vi "PDash Duplicate Module.vi"(8 "error in":errorcluster, 10 "Current Selection":T1, 11 "Project":refnum<class "Project.lvclass">) -> (0 "error out":errorcluster)   [LabVIEW 2020, in "Panther Dashboard.lvlib"]
doc: "Panther Dashboard DQMH UI Template"
uses:
  Panther Dashboard.lvlib
  Class/Project/Project.lvclass
  Class/Library/Library.lvclass
  C:/GitClones/PantherLAB/PantherDashboard/src/LabVIEW/Panther Dashboard/Class/LabVIEWItem/LabVIEWItem.lvclass
  Class/VI/VI.lvclass
  Class/Library/Library.lvclass/Library.ctl
  Class/LabVIEWItem/LabVIEWItem.lvclass/LabVIEWItem.ctl
  Class/Project/Project.lvclass/Project.ctl
  <vilib>/Delacor/Delacor QMH/Libraries/_Scripting Support/Module Type--enum.ctl
  <vilib>/Delacor/Delacor QMH/Libraries/_Scripting Support/dqmh_lib_DQMH Scripting Support.lvlib
  <vilib>/Delacor/Delacor QMH/Libraries/_Scripting Support/Module Info--cluster.ctl
  Controls/Cancel.ctl
  Controls/Continue.ctl
panel:
  out "Selected Module":string caption="Current Module Selection:"
  in  "Module Description":string caption="New Module Description"
  in  "New Module Path":path
  in  "Module Name":string caption="New Module Name"
  in  "Continue":T2
  in  "Cancel":T3
  # "Note: To Select the DQMH Default UIs, click the Gear Icon on the Panther Dashboard\nMain UI, and Uncheck the 'Use Panther Dashboard UIs' checkbox."
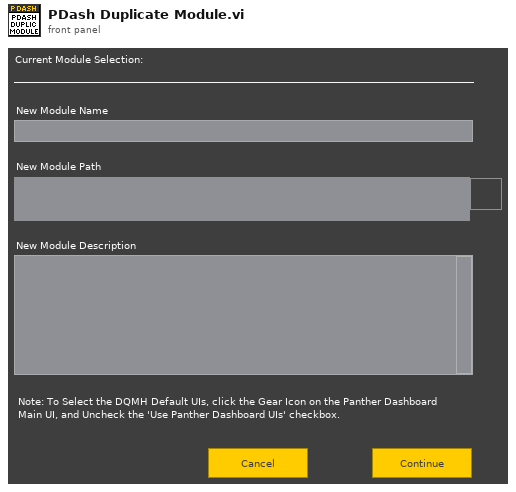
[diagram p1: front panel]
types:
  T1 = cluster{"Library":refnum<class "Library.lvclass">, "VI":refnum<class "VI.lvclass">}
  T2 = typedef "Continue.ctl" = bool
  T3 = typedef "Cancel.ctl" = bool
  T4 = typedef "dqmh_lib_DQMH Scripting Support.lvlib/Module Info--cluster.ctl" = cluster{"Name":string, "Library":refnum<vi>, "Library Owning App":refnum<vi>, "Library Owning Folder":path, "Module Type":T5, "Public API Requests Folder":refnum<vi>, "Public API Requests Arguments Folder":refnum<vi>, "Broadcasts Folder":refnum<vi>, "Broadcasts Arguments Folder":refnum<vi>, "Obtain Broadcast Events VI":refnum<vi>, "Destroy Broadcast Events VI":refnum<vi>, "Obtain Request Events VI":refnum<vi>, "Destroy Request Events VI":refnum<vi>, "Request Events Cluster CTL":refnum<vi>, "Broadcast Events Cluster CTL":refnum<vi>, "Module Timeout VI":refnum<vi>, "Module Name VI":refnum<vi>, "Status Updated VI":refnum<vi>, "Module Not Running Error Constant VI":refnum<vi>}
  T5 = typedef "dqmh_lib_DQMH Scripting Support.lvlib/Module Type--enum.ctl" = enum16{"Singleton", "Cloneable"}
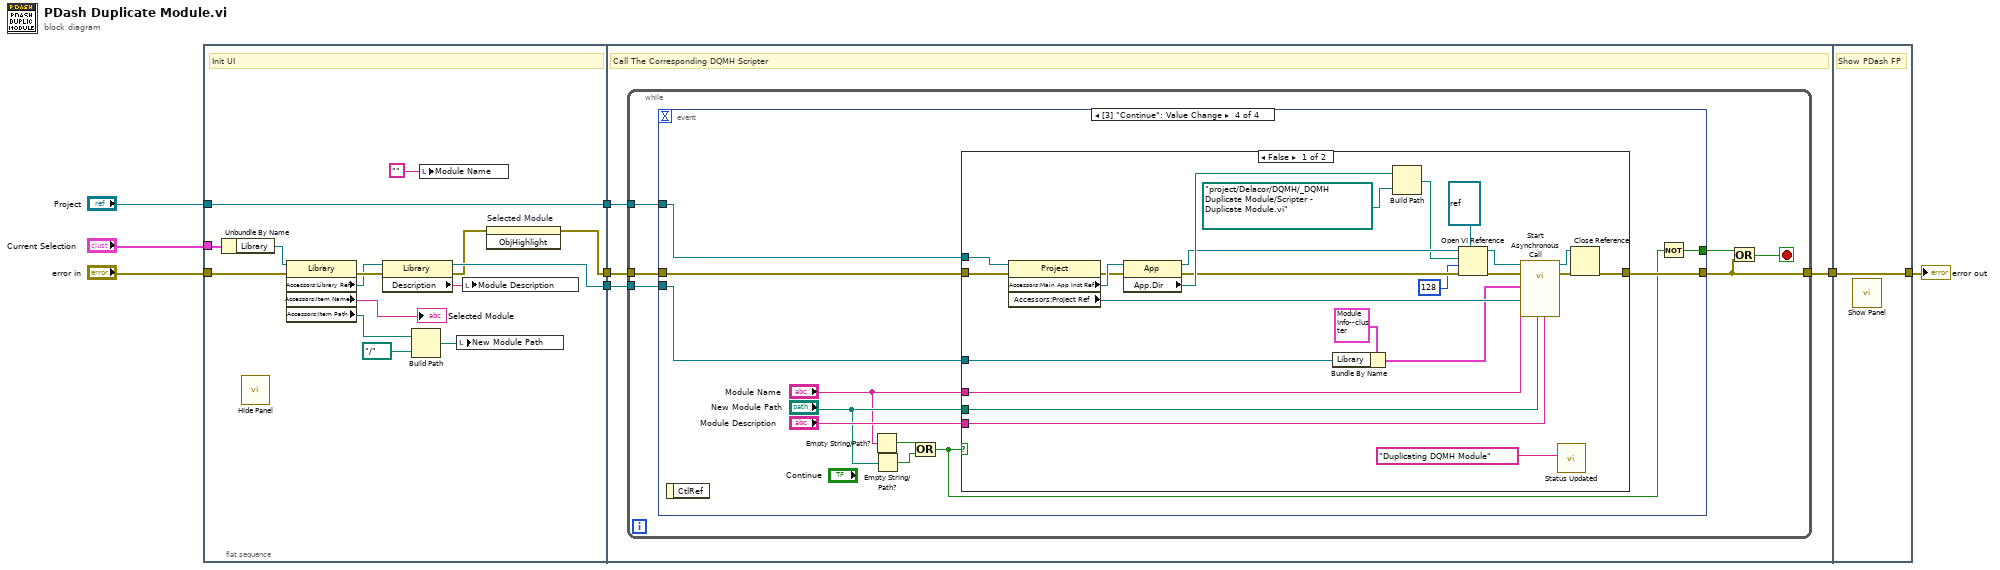
[diagram p0: block diagram]
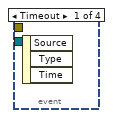
[diagram p2: hidden frame]
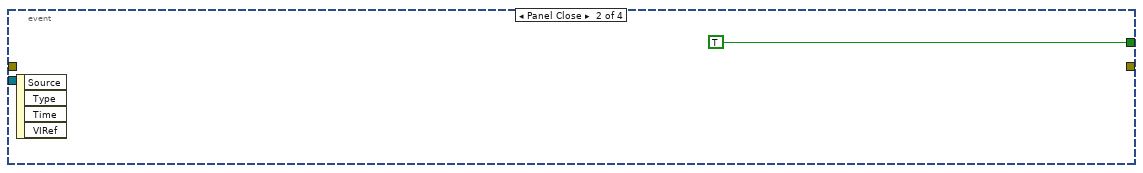
[diagram p3: hidden frame]
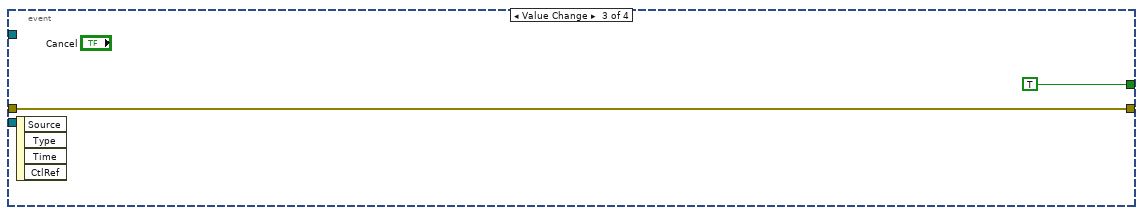
[diagram p4: hidden frame]
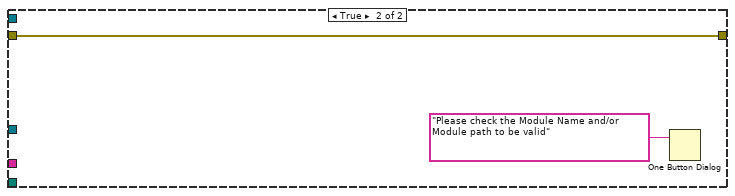
[diagram p5: hidden frame]
diagram:
  n1 = flat-sequence {
    tunnel: "Project" -> [w21]
    tunnel: [w21] -> w3
    tunnel: "error in" -> [w23]
    tunnel: [w9] -> w5
    tunnel: "Current Selection" -> [w20]
    tunnel: [w13] -> w1
    tunnel: [w27] -> w8
    tunnel: w3 -> [w25]
    tunnel: w5 -> [w26]
    tunnel: w1 -> [w24]
    tunnel: [w74] -> w7
    tunnel: w8 -> [w74]
    frame #0 {
      # "Init UI"
      n2 = Unbundle By Name(w20) -> ("Library"=w19:refnum<class "Library.lvclass">)
      n3 = call "Hide Panel.vi"() -> ()  [unwired: 11 in, 1 out]
      n4 = property class="Library"(reference=w19, error in=w23) -> (error out=w22:errorcluster, "Accessors:Library Ref"=w14:refnum<vi>, "Accessors:Item Name"=→"Selected Module":string, "Accessors:Item Path"=w16:path)  [unwired: 1 out]
      n5 = property class="Library"(reference=w14, error in=w22) -> (reference out=w13:refnum<vi>, error out=w10:errorcluster, "Description"=w12:string)
      n6 = Build Path(base path=w16, name or relative path=path "../..") -> (appended path=w18:path)
      n7 = local write "Module Name"("") -> ()
      n8 = local write "New Module Path"(w18) -> ()
      n9 = local write "Module Description"(w12) -> ()
      n10 = invoke on="Selected Module" class="Str" method="ObjHighlight"(error in=w10) -> (error out=w9:errorcluster)  [unwired: 2 in, 2 out]
    }
    frame #1 {
      # "Call The Corresponding DQMH Scripter"
      n11 = while {
        tunnel: [w28] -> w27
        tunnel: w25 -> [w31]
        tunnel: w26 -> [w33]
        tunnel: w24 -> [w30]
        stop <- w29 stop-if-true
        n12 = event shown="[3] \"Continue\": Value Change" {
          selector: _ -> [_ _ _ _]
          dyn-events: _ -> [_ _ _ _]
          timeout: _ -> [_ _ _ _]
          tunnel: [_ TRUE TRUE w45] -> w32
          tunnel: [_ _ w35 w38] -> w28
          tunnel: w31 -> [_ _ _ w41]
          tunnel: w33 -> [_ _ w35 w40]
          tunnel: w30 -> [_ _ _ w39]
          event Timeout {
            n13 = event-data() -> ()  [unwired: 1 in, 3 out]
          }
          event Panel Close {
            n14 = event-data() -> ()  [unwired: 1 in, 4 out]
          }
          event Value Change {
            n15 = event-data() -> ()  [unwired: 1 in, 4 out]
          }
          event Value Change {
            n16 = event-data() -> ()  [unwired: 1 in, 1 out]
            n17 = Empty String/Path?(string/path="Module Name") -> (empty?=w47:bool)
            n18 = Empty String/Path?(string/path="New Module Path") -> (empty?=w46:bool)
            n19 = Or(x=w47, y=w46) -> (x .or. y?=w37:bool)
            n20 = case shown="False" w37 {
              tunnel: "Module Description" -> [w58 _]
              tunnel: "New Module Path" -> [w57 _]
              tunnel: "Module Name" -> [w56 _]
              tunnel: w41 -> [w55 _]
              tunnel: w40 -> [w54 w72]
              tunnel: w39 -> [w52 _]
              tunnel: [w48 w72] -> w38
              frame False {
                n21 = property class="Project"(reference=w55, error in=w54) -> (error out=w62:errorcluster, "Accessors:Main App Inst Ref"=w68:refnum<vi>, "Accessors:Project Ref"=w69:refnum<vi>)  [unwired: 1 out]
                n22 = property class="App"(reference=w68, error in=w62) -> (reference out=w66:refnum<vi>, error out=w61:errorcluster, "App.Dir"=w67:path)
                n23 = Bundle By Name(cluster=T4 {"Name"="", "Library"=refnum, "Library Owning App"=refnum, "Library Owning Folder"=path "", "Module Type"=enum."Singleton", "Public API Requests Folder"=refnum, "Public API Requests Arguments Folder"=refnum, "Broadcasts Folder"=refnum, "Broadcasts Arguments Folder"=refnum, "Obtain Broadcast Events VI"=refnum, "Destroy Broadcast Events VI"=refnum, "Obtain Request Events VI"=refnum, "Destroy Request Events VI"=refnum, "Request Events Cluster CTL"=refnum, "Broadcast Events Cluster CTL"=refnum, "Module Timeout VI"=refnum, "Module Name VI"=refnum, "Status Updated VI"=refnum, "Module Not Running Error Constant VI"=refnum} ("Module Info in"), "Library"=w52) -> (w64:T4)
                n24 = Build Path(base path=w67, name or relative path=path "project/Delacor/DQMH/_DQMH Duplicate Module/Scripter - Duplicate Module.vi") -> (appended path=w63:path)
                n25 = Open VI Reference(type specifier VI Refnum (for type only)=refnum<vi> refnum, application reference (local)=w66, vi path=w63, options=128, error in (no error)=w61) -> (vi reference=w70:refnum<vi>, error out=w59:errorcluster)  [unwired: 1 in]
                n26 = call-by-ref "Start Asynchronous Call"(reference=w70, error in=w59, "Description"=w58, "Save Folder"=w57, "Project"=w69, "New Module Name"=w56, "Module Info in"=w64) -> (reference out=w65:refnum<vi>, error out=w60:errorcluster)  [unwired: 5 in, 2 out]
                n27 = call "Status Updated.vi"("Status"="Duplicating DQMH Module") -> ()  [unwired: 10 in, 1 out]
                n28 = Close Reference(reference=w65, error in (no error)=w60) -> (error out=w48:errorcluster)
              }
              frame True {
                n29 = One Button Dialog(message="Please check the Module Name and/or Module path to be valid") -> ()  [unwired: 1 in, 1 out]
              }
            }
            n30 = Not(x=w37) -> (.not. x?=w45:bool)
          }
        }
        n31 = Or(x=w32, y=w28) -> (x .or. y?=w29:bool)
      }
    }
    frame #2 {
      # "Show PDash FP"
      n32 = call "Show Panel.vi"() -> ()  [unwired: 11 in, 1 out]
    }
  }
  "error out" <- w7
